vi "AMC Error Pause Stop Exit.vi"(8 "error in (no error)":errorcluster, 11 "Message Queue In":T1) -> (0 "error out":errorcluster, 3 "Message Queue Out":T1)   [LabVIEW 2017]
uses:
  subVIs/TypeDefs/amc_Message Queue.ctl
  subVIs/TypeDefs/amc_Message.ctl
  Tools/Keyed Array/Tools_KeyedArray KeyedArray.ctl
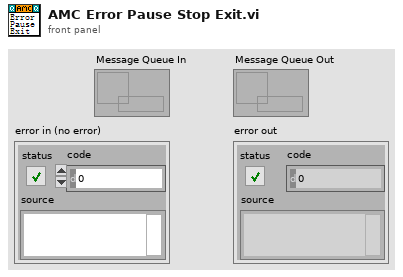
[diagram p1: front panel]
types:
  T1 = typedef "amc_Message Queue.ctl" = refnum<queue>
  T2 = cluster{"1 Number":i32, "2 Number":i32, "3 Number":i32}
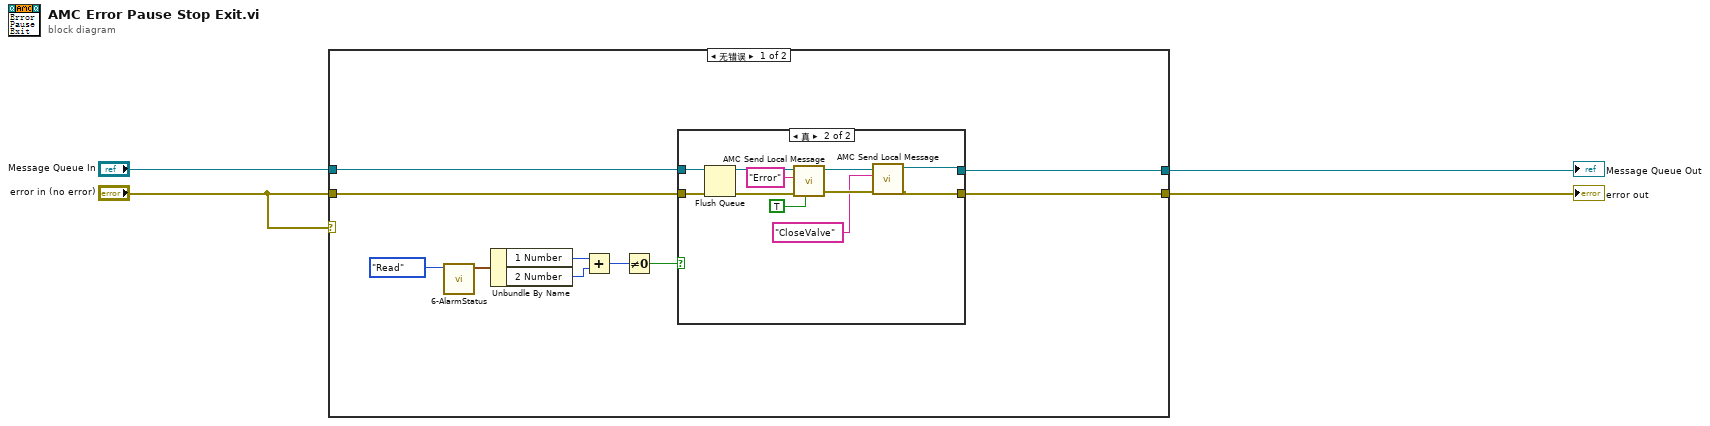
[diagram p0: block diagram]
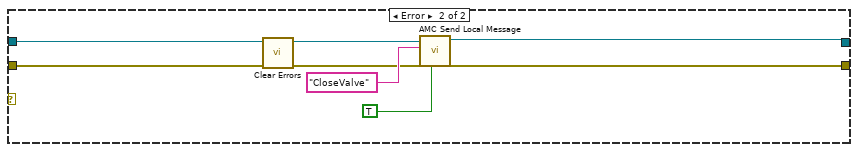
[diagram p3: hidden frame]
diagram:
  n1 = case shown="无错误" "error in (no error)" {
    tunnel: "Message Queue In" -> [w8 w31]
    tunnel: [w7 w30] -> w3
    tunnel: "error in (no error)" -> [w6 w28]
    tunnel: [w5 w29] -> w2
    frame No Error {
      n2 = call "6-AlarmStatus.vi"("Step"=enum16{"Initial", "Write", "Read"}."Read") -> ("AlarmNumber"=w13:T2)  [unwired: 8 in, 2 out]
      n3 = Unbundle By Name(w13) -> ("1 Number"=w12:i32, "2 Number"=w11:i32)
      n4 = Add(x=w12, y=w11) -> (x+y=w10:i32)
      n5 = Not Equal To 0?(x=w10) -> (x != 0?=w9:bool)
      n6 = case shown="真" w9 {
        tunnel: w8 -> [w16 w25]
        tunnel: [w16 w20] -> w7
        tunnel: w6 -> [w15 w24]
        tunnel: [w15 w19] -> w5
        frame False {
        }
        frame True {
          n7 = Flush Queue(queue=w25) -> (queue out=w22:T1)  [unwired: 1 in, 2 out]
          n8 = call "AMC Send Local Message.vi"("Priority Message (F)"=TRUE, "error in (no error)"=w24, "Message Name"="Error", "Message Queue in"=w22) -> ("error out"=w18:errorcluster, "Message Queue out"=w21:T1)  [unwired: 6 in]
          n9 = call "AMC Send Local Message.vi"("error in (no error)"=w18, "Message Name"="CloseValve", "Message Queue in"=w21) -> ("error out"=w19:errorcluster, "Message Queue out"=w20:T1)  [unwired: 7 in]
        }
      }
    }
    frame Error {
      n10 = call <vilib>:"Clear Errors.vi"("error in (no error)"=w28) -> ("error out"=w27:errorcluster)  [unwired: 5 in, 1 out]
      n11 = call "AMC Send Local Message.vi"("Priority Message (F)"=TRUE, "error in (no error)"=w27, "Message Name"="CloseValve", "Message Queue in"=w31) -> ("error out"=w29:errorcluster, "Message Queue out"=w30:T1)  [unwired: 6 in]
    }
  }
  "Message Queue Out" <- w3
  "error out" <- w2
